vi "UDP Connection Handler.vi"(8 "Chunks To Send":refnum<notifier>, 9 "TCP Connection":refnum<k5>, 10 "Remote Address":string) -> ()   [LabVIEW 2017]
panel:
  out "Local UDP Port":u16
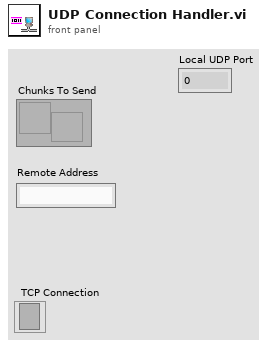
[diagram p1: front panel]
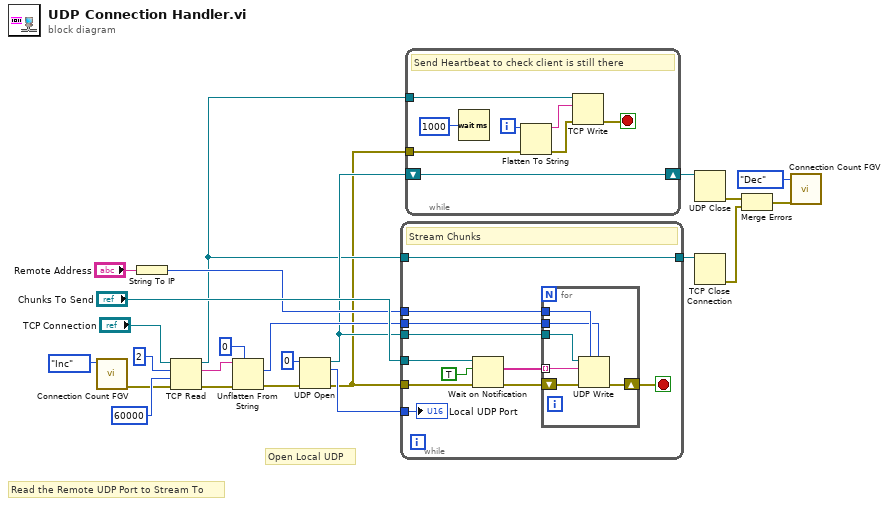
[diagram p0: block diagram]
diagram:
  # "Open Local UDP"
  # "Read the Remote UDP Port to Stream To"
  n1 = call "Connection Count FGV.vi"("Action (Read)"=enum16{"Read", "Inc", "Dec"}."Inc") -> ("error out"=w3:errorcluster)  [unwired: 9 in, 1 out]
  n2 = String To IP(1:"Remote Address") -> (0:w22:u32)
  n3 = TCP Read(connection ID="TCP Connection", bytes to read=2, error in (no error)=w3, 9:60000 ("timeout ms (25000)")) -> (connection ID out=w8:refnum<k5>, data out=w16:string, error out=w14:errorcluster)  [unwired: 1 in]
  n4 = Unflatten From String(type=u16 0 ("Remote Port"), binary string=w16, error in (no error)=w14) -> (value=w11:u16, error out=w12:errorcluster)  [unwired: 2 in, 1 out]
  n5 = UDP Open(8:w12, 11:u16 0 ("port")) -> (port=w10:refnum<k16>, 0:w1:errorcluster, 2:w2:u16)  [unwired: 3 in]
  n6 = while {
    tunnel: "Chunks To Send" -> [w35]
    tunnel: w22 -> [w34]
    tunnel: w10 -> [w33]
    tunnel: w11 -> [w29]
    tunnel: w8 -> [w27]
    tunnel: [w27] -> w7
    tunnel: w2 -> [w26]
    tunnel: w1 -> [w25]
    stop <- w28 stop-if-true
    # "Stream Chunks"
    n7 = Wait on Notification(notifier=w35, ignore previous (F)=TRUE, error in (no error)=w25) -> (notification=w31:string[], error out=w30:errorcluster)  [unwired: 1 in, 2 out]
    n8 = for {
      tunnel: w31 -> [w41] mode=indexing
      tunnel: w34 -> [w40]
      shift-right: [w39] -> w28
      shift-left: w30 -> [w38]
      tunnel: w33 -> [w37]
      tunnel: w29 -> [w36]
      n9 = UDP Write(address=w40, port or service name=w36, connection ID=w37, data in=w41, 8:w38) -> (error out=w39:errorcluster)  [unwired: 1 in, 1 out]
    }
    "Local UDP Port" <- w26
  }
  n10 = while {
    tunnel: w8 -> [w49]
    shift-right: [w45] -> w9
    shift-left: w10 -> [w45]
    tunnel: w1 -> [w43]
    i -> [w42]
    stop <- w47 stop-if-true
    # "Send Heartbeat to check client is still there"
    n11 = Wait (ms)(milliseconds to wait=u32 1000) -> ()  [unwired: 1 out]
    n12 = Flatten To String(anything=w42, error in (no error)=w43) -> (data string=w46:string, error out=w44:errorcluster)  [unwired: 2 in, 1 out]
    n13 = TCP Write(connection ID=w49, data in=w46, error in (no error)=w44) -> (error out=w47:errorcluster)  [unwired: 1 in, 2 out]
  }
  n14 = UDP Close(connection ID=w9) -> (error out=w6:errorcluster)  [unwired: 1 in, 1 out]
  n15 = TCP Close Connection(connection ID=w7) -> (error out=w5:errorcluster)  [unwired: 2 in, 1 out]
  n16 = Merge Errors(w6, w5) -> (w4:errorcluster)
  n17 = call "Connection Count FGV.vi"("error in (no error)"=w4, "Action (Read)"=enum16{"Read", "Inc", "Dec"}."Dec") -> ()  [unwired: 8 in, 2 out]
